vi "WFDC Compute Z Calibration.vi"(0 "Scan Positions File Name":string="Scan Positions.xml", 1 "User Close?":bool=TRUE, 2 "Half Shift":i32=7, 7 "Data Path":path, 11 "Error":errorcluster) -> (4 "Fit Slope":dbl=0.02 format="%#_6f", 8 "Fit Intercept":dbl=0.02, 13 "Ref Images":T1[](array[typedef]), 15 "Error":errorcluster)   [LabVIEW 2016]
uses:
  <vilib>/vision/Image Controls.llb/IMAQ Image.ctl
  WFDC Controls/WFDC Reference Image Info.ctl
  <vilib>/Utility/miscctls.llb/LVPointTypeDef.ctl
  <vilib>/Analysis/6fits.llb/Curve Fitting Criteria.ctl
  WFDC DLL and Testing/Visual Studio NCC Max Shift DLL/x64/Release/VSmaxShiftNCC.dll
  <vilib>/Analysis/NI_AALPro.lvlib
panel:
  out "Z Calibration":cluster{dbl[], dbl[]}[](graph)
  in  "Done":bool
  out "Wait Bar":i32(slide) scale=0.0..11.0
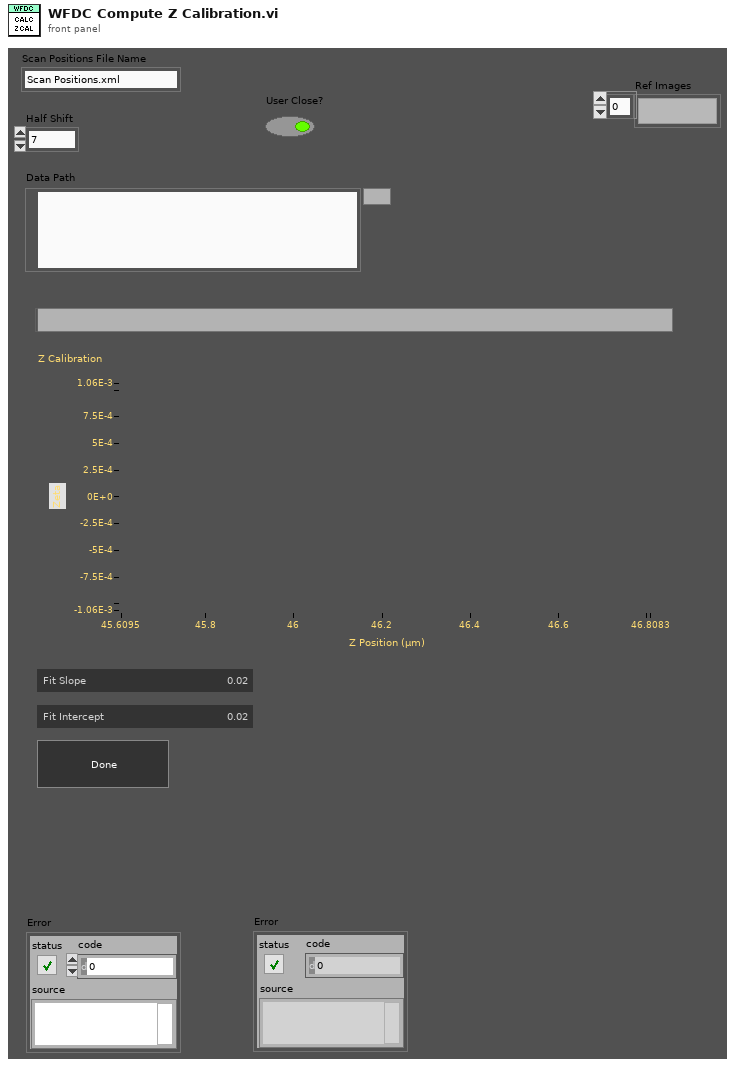
[diagram p1: front panel]
types:
  T1 = typedef "IMAQ Image.ctl" = refnum<image>
  T2 = enum16{"Always On", "Always Off", "Off While Running"}
  T3 = typedef "LVPointTypeDef.ctl" = cluster{"Horizontal":i16, "Vertical":i16}
  T4 = typedef "WFDC Reference Image Info.ctl" = cluster{"Image Path":path, "Z Position":dbl, "Number of Frames":u32}
  T5 = typedef "LVRectTypeDef.ctl" = cluster{"Left":i16, "Top":i16, "Right":i16, "Bottom":i16}
  T6 = typedef "LVBoundsTypeDef.ctl" = cluster{"Width":u32, "Height":u32}
  T7 = typedef "NI_AALPro.lvlib/Curve Fitting Criteria.ctl" = u16
  T8 = typedef "TIF Read Image Information.ctl" = cluster{"Byte Order":enum16{"big-endian, network order", "native, host order", "little-endian"}, "Width (pixels)":i32, "Height (pixels)":i32, "Bits per Pixel":u8, "Total Frames":u32, "First Frame Offset (bytes)":u32, "Frame Size (bytes)":u32}
  T9 = typedef "Image Type" = u32
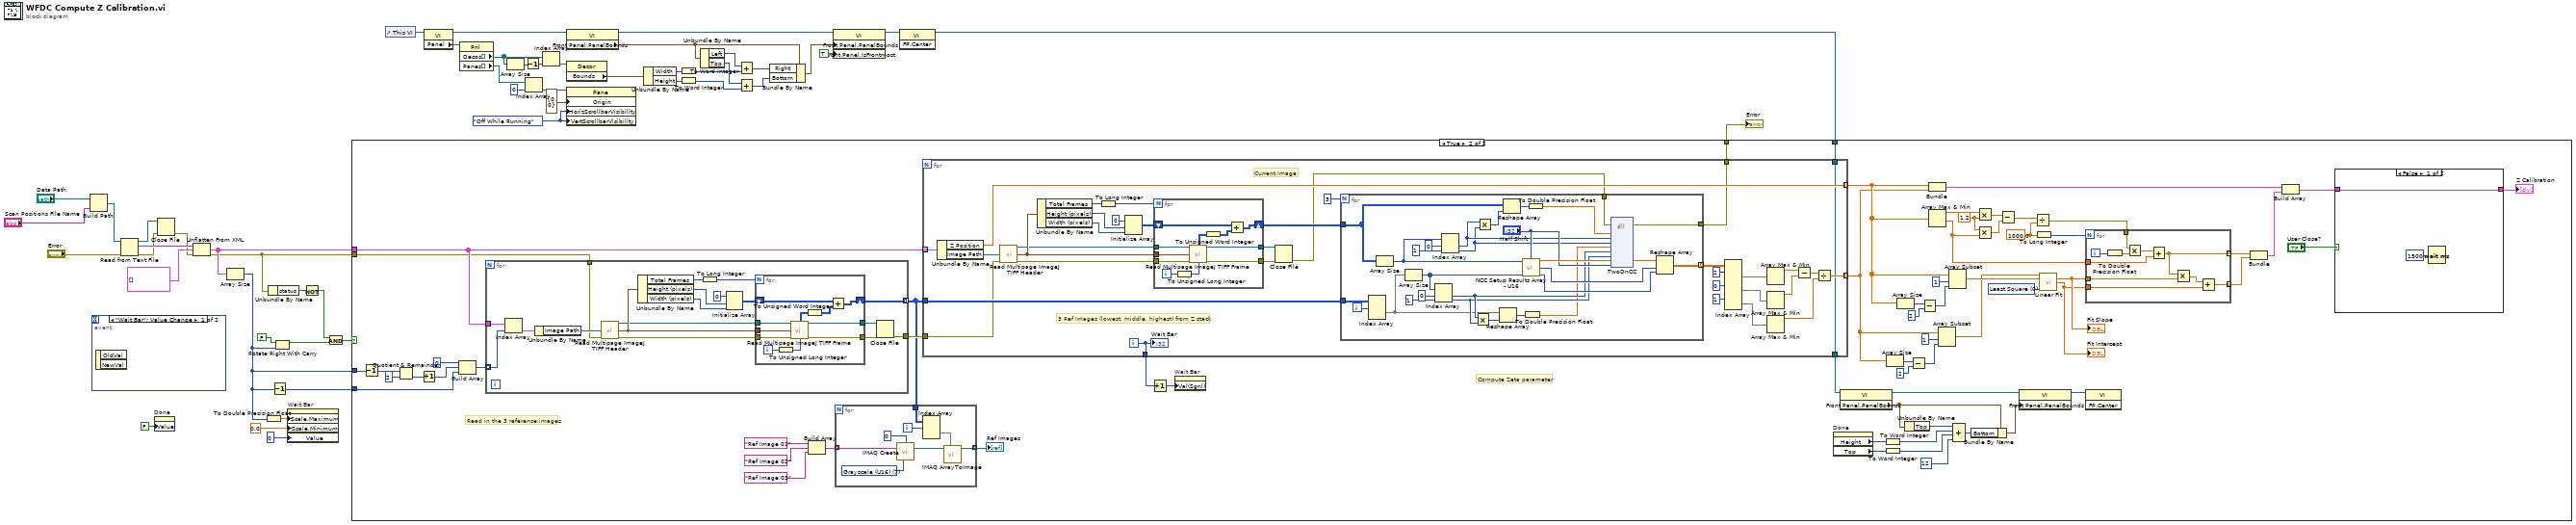
[diagram p0: block diagram]
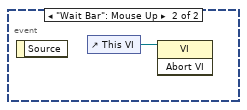
[diagram p2: hidden frame]
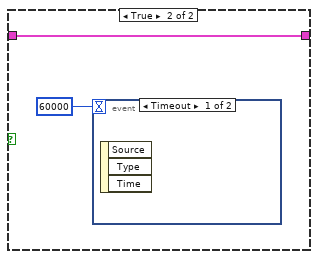
[diagram p4: hidden frame]
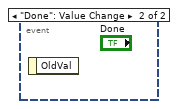
[diagram p5: hidden frame]
diagram:
  w25 = T2."Off While Running" ("Vertical Scrollbar Visibility")
  n1 = Build Path(base path="Data Path", name or relative path="Scan Positions File Name") -> (appended path=w1:path)
  n2 = event shown="[0] \"Wait Bar\": Value Change" {
    selector: _ -> [_ _]
    dyn-events: _ -> [_ _]
    timeout: _ -> [_ _]
    event "Wait Bar": Value Change {
      n3 = event-data() -> ()  [unwired: 1 in, 2 out]
    }
    event "Wait Bar": Mouse Up {
      n4 = event-data() -> ()  [unwired: 1 in, 1 out]
      n5 = control-ref of="This VI"() -> (w51:refnum<vi>)
      n6 = invoke class="VI" method="Abort VI"(reference=w51) -> ()  [unwired: 2 in, 3 out]
    }
  }
  n7 = Read from Text File(file (use dialog)=w1, error in="Error") -> (refnum out=w49:refnum<file>, text=w50:string, error out=w44:errorcluster)  [unwired: 2 in, 1 out]
  n8 = property on="Done" class="Bool (strict)"("Value"=FALSE ("Done")) -> ()  [unwired: 2 in, 2 out]
  n9 = Close File(refnum=w49, error in=w44) -> (error out=w43:errorcluster)  [unwired: 1 out]
  n10 = Unflatten From XML(xml string=w50, type=T4[] [], error in (no error)=w43) -> (value=w46:T4[], error out=w42:errorcluster)
  n11 = Array Size(array=w46) -> (size(s)=w9:i32)
  n12 = To Double Precision Float(number=w9) -> (double precision float=w8:dbl)
  n13 = Unbundle By Name(w42) -> ("status"=w41:bool)
  n14 = Decrement(x=w9) -> (x-1=w45:i32)
  n15 = Rotate Right With Carry(2:w9, 3:FALSE ("carry")) -> (1:w39:bool)  [unwired: 1 out]
  n16 = property on="Wait Bar" class="Slide (strict)"("Scale.Maximum"=w8, "Scale.Minimum"=0.0 ("Scale.Range:Minimum"), "Value"=0 ("Wait Bar")) -> ()  [unwired: 2 in, 2 out]
  n17 = Not(x=w41) -> (.not. x?=w40:bool)
  n18 = And(x=w40, y=w39) -> (x .and. y?=w38:bool)
  n19 = control-ref of="This VI"() -> (w12:refnum<vi>)
  n20 = property class="VI"(reference=w12) -> (reference out=w26:refnum<vi>, "Panel"=w19:refnum<vi>)  [unwired: 1 in, 1 out]
  n21 = property class="Pnl"(reference=w19) -> ("Decos[]"=w18:refnum<vi>[], "Panes[]"=w22:refnum<vi>[])  [unwired: 1 in, 2 out]
  n22 = Array Size(array=w18) -> (size(s)=w16:i32)
  n23 = Decrement(x=w16) -> (x-1=w17:i32)
  n24 = Index Array(array=w22, index=0) -> (element=w21:refnum<vi>)
  n25 = Index Array(array=w18, index=w17) -> (element=w24:refnum<vi>)
  n26 = property class="VI"(reference=w26) -> (reference out=w28:refnum<vi>, "Front Panel.PanelBounds"=w29:T5)  [unwired: 1 in, 1 out]
  n27 = property class="Decor"(reference=w24) -> ("Bounds"=w27:T6)  [unwired: 1 in, 2 out]
  n28 = property class="Pane"(reference=w21, "Origin"=T3 {"Horizontal"=0, "Vertical"=0}, "HorizScrollbarVisibility"=w25, "VertScrollbarVisibility"=w25) -> ()  [unwired: 1 in, 2 out]
  n29 = Unbundle By Name(w27) -> ("Width"=w32:u32, "Height"=w35:u32)
  n30 = To Word Integer(number=w32) -> (16bit integer=w34:i16)
  n31 = To Word Integer(number=w35) -> (16bit integer=w13:i16)
  n32 = Unbundle By Name(w29) -> ("Left"=w31:i16, "Top"=w15:i16)
  n33 = Add(x=w31, y=w34) -> (x+y=w33:i16)
  n34 = Add(x=w15, y=w13) -> (x+y=w14:i16)
  n35 = Bundle By Name(cluster=w29, "Right"=w33, "Bottom"=w14) -> (w30:T5)
  n36 = property class="VI"(reference=w28, "Front Panel.PanelBounds"=w30, "Front Panel.IsFrontmost"=TRUE ("Front Panel Window:Is Frontmost")) -> (reference out=w5:refnum<vi>)  [unwired: 1 in, 1 out]
  n37 = invoke class="VI" method="FP.Center"(reference=w5) -> (reference out=w4:refnum<vi>)  [unwired: 2 in, 2 out]
  n38 = case shown="True" w38 {
    tunnel: w9 -> [_ w116]
    tunnel: w46 -> [_ w108]
    tunnel: w45 -> [_ w110]
    tunnel: w42 -> [w52 w81]
    tunnel: [w52 w79] -> w36
    tunnel: w4 -> [_ w74]
    frame False {
    }
    frame True {
      w101 = 1000.0 ("y")
      w105 = 1.2 ("y")
      w107 = T7 0 items=["Least Square", "Least Absolute Residual", "Bisquare"] ("method")
      # "Compute Zeta parameter"
      # "Read in the 3 reference images"
      n39 = Decrement(x=w116) -> (x-1=w115:i32)
      n40 = Quotient & Remainder(x=w115, y=2) -> (floor(x/y)=w113:i32)  [unwired: 1 out]
      n41 = Increment(x=w113) -> (x+1=w112:i32)
      n42 = Build Array(0 ("element"), w112, w110) -> (w109:i32[])
      n43 = for {
        tunnel: w109 -> [w228] mode=indexing
        tunnel: w108 -> [w229]
        tunnel: [w215] -> w60 mode=indexing
        tunnel: [w213] -> w80
        tunnel: w81 -> [w212]
        n44 = Index Array(array=w229, index=w228) -> (element=w227:T4)
        n45 = Unbundle By Name(w227) -> ("Image Path"=w216:path)
        n46 = call "Read Multipage ImageJ TIFF Header.vi"("TIFF Path"=w216, "Error"=w212) -> ("TIF Ref"=w218:refnum<file>, "Image Info"=w220:T8, "Error"=w219:errorcluster)  [unwired: 11 in]
        n47 = Unbundle By Name(w220) -> ("Total Frames"=w221:u32, "Height (pixels)"=w225:i32, "Width (pixels)"=w224:i32)
        n48 = To Long Integer(number=w221) -> (32bit integer=w222:i32)
        n49 = Initialize Array(u16 0 ("element"), w225, w224) -> (w223:u16[][])
        n50 = for {
          N: w222 -> [_]
          tunnel: w218 -> [w240]
          tunnel: w220 -> [w239]
          tunnel: w219 -> [w238]
          shift-right: [w234] -> w215
          shift-left: w223 -> [w235]
          tunnel: [w233] -> w226
          tunnel: [w232] -> w214
          i -> [w237]
          n51 = To Unsigned Long Integer(number=w237) -> (unsigned 32bit integer=w236:u32)
          n52 = call "Read Multipage ImageJ TIFF Frame.vi"("TIF Ref"=w240, "Image Info"=w239, "Error"=w238, "Frame"=w236) -> ("U8 Image"=w231:u8[][], "TIF Ref (Dup)"=w233:refnum<file>, "Error"=w232:errorcluster)  [unwired: 8 in, 1 out]
          n53 = To Unsigned Word Integer(number=w231) -> (unsigned 16bit integer=w230:u16[][])
          n54 = Add(x=w235, y=w230) -> (x+y=w234:u16[][])
        }
        n55 = Close File(refnum=w226, error in=w214) -> (error out=w213:errorcluster)  [unwired: 1 out]
      }
      n56 = Build Array("Ref Image 01" ("Image Name"), "Ref Image 02" ("Image Name"), "Ref Image 03" ("Image Name")) -> (w64:string[])
      n57 = for {
        tunnel: w64 -> [w126] mode=indexing
        tunnel: w60 -> [w124]
        tunnel: [w121] -> w59 mode=indexing
        i -> [w122]
        w127 = T9 7 items=["Grayscale (U8)", "Grayscale (I16)", "Grayscale (SGL)", "Complex (CSG)", "RGB (U32)", "HSL (U32)", "RGB (U64)", "Grayscale (U16)"] ("Image Type")
        n58 = call "IMAQ Create"("Border Size"=0, "Image Name"=w126, "Image Type"=w127) -> ("New Image"=w125:T1)  [unwired: 2 in, 1 out]
        n59 = Index Array(array=w124, index (dim 0)=w122) -> (element=w123:u16[][])  [unwired: 2 in]
        n60 = call "IMAQ ArrayToImage"("Image Pixels (U16)"=w123, "Image"=w125) -> ("Image Out"=w121:T1)  [unwired: 8 in, 1 out]
      }
      "Ref Images" <- w59
      n61 = for {
        tunnel: w60 -> [w172]
        tunnel: w108 -> [w171] mode=indexing
        tunnel: [w170] -> w83 mode=indexing
        tunnel: [w169] -> w82 mode=indexing
        tunnel: w80 -> [w168]
        tunnel: [w167] -> w79
        tunnel: [w166] -> w78
        tunnel: w74 -> [w165]
        tunnel: [w165] -> w73
        i -> [w166]
        # "Current Image"
        # "3 Ref Images (lowest, middle, highest) from Z stack"
        n62 = Unbundle By Name(w171) -> ("Z Position"=w170:dbl, "Image Path"=w154:path)
        n63 = call "Read Multipage ImageJ TIFF Header.vi"("TIFF Path"=w154, "Error"=w168) -> ("TIF Ref"=w156:refnum<file>, "Image Info"=w158:T8, "Error"=w157:errorcluster)  [unwired: 11 in]
        n64 = Unbundle By Name(w158) -> ("Total Frames"=w159:u32, "Height (pixels)"=w163:i32, "Width (pixels)"=w162:i32)
        n65 = To Long Integer(number=w159) -> (32bit integer=w160:i32)
        n66 = Initialize Array(u16 0 ("element"), w163, w162) -> (w161:u16[][])
        n67 = for {
          N: w160 -> [_]
          tunnel: w156 -> [w211]
          tunnel: w158 -> [w210]
          tunnel: w157 -> [w209]
          shift-right: [w205] -> w152
          shift-left: w161 -> [w206]
          tunnel: [w204] -> w164
          tunnel: [w203] -> w140
          i -> [w208]
          n68 = To Unsigned Long Integer(number=w208) -> (unsigned 32bit integer=w207:u32)
          n69 = call "Read Multipage ImageJ TIFF Frame.vi"("TIF Ref"=w211, "Image Info"=w210, "Error"=w209, "Frame"=w207) -> ("U8 Image"=w202:u8[][], "TIF Ref (Dup)"=w204:refnum<file>, "Error"=w203:errorcluster)  [unwired: 8 in, 1 out]
          n70 = To Unsigned Word Integer(number=w202) -> (unsigned 16bit integer=w201:u16[][])
          n71 = Add(x=w206, y=w201) -> (x+y=w205:u16[][])
        }
        n72 = Close File(refnum=w164, error in=w140) -> (error out=w139:errorcluster)  [unwired: 1 out]
        n73 = for {
          N: 3 -> [_]
          tunnel: w172 -> [w200]
          tunnel: w152 -> [w180]
          tunnel: [w175] -> w151 mode=indexing
          tunnel: w139 -> [w174]
          tunnel: [w173] -> w167
          i -> [w199]
          n74 = Index Array(array=w200, index (dim 0)=w199) -> (element=w187:u16[][])  [unwired: 2 in]
          n75 = Array Size(array=w180) -> (size(s)=w182:i32[])
          n76 = Array Size(array=w187) -> (size(s)=w193:i32[])
          n77 = Index Array(array=w193, index #1=0 ("index"), index #2=1 ("index")) -> (element #1=w190:i32, element #2=w189:i32)
          n78 = Index Array(array=w182, index #1=0 ("index"), index #2=1 ("index")) -> (element #1=w178:i32, element #2=w177:i32)
          n79 = Multiply(x=w190, y=w189) -> (x*y=w188:i32)
          n80 = Multiply(x=w178, y=w177) -> (x*y=w176:i32)
          n81 = Reshape Array(w187, w188) -> (w186:u16[])
          n82 = Reshape Array(w180, w176) -> (w181:u16[])
          n83 = call "NCC Setup Results Array - U16.vi"("Image 01 Size"=w182, "Half Shift"="Half Shift", "Image 02 Size"=w193) -> ("NCC Results Array"=w198:dbl[], "Result Rows"=w195:i32, "Result Columns"=w196:i32)  [unwired: 10 in]
          n84 = To Double Precision Float(number=w186) -> (double precision float=w185:dbl[])
          n85 = To Double Precision Float(number=w181) -> (double precision float=w179:dbl[])
          n86 = dll-call lib="C:/Users/George Sirinakis/Documents/Microscope-Control/Microscope Modules/Wide Field Drift Correction/WFDC DLL and Testing/Visual Studio NCC Max Shift DLL/x64/Release/VSmaxShiftNCC.dll" fn="TwoDnCC"(error in=w174, "im01"=w179, "im01rowSize"=w178, "im01colSize"=w177, "im02"=w185, "im02rowSize"=w190, "im02ColSize"=w189, "theResult"=w198, "halfShift"="Half Shift") -> (error out=w173:errorcluster, "theResult"=w197:dbl[])  [unwired: 10 in, 1 out]
          n87 = Reshape Array(w197, w195, w196) -> (w175:dbl[][])
        }
        n88 = Index Array(array=w151, index (dim 0) #1=2 ("index (page)"), index (dim 0) #2=0 ("index (page)"), index (dim 0) #3=1 ("index (page)")) -> (element #1=w143:dbl[][], element #2=w141:dbl[][], element #3=w142:dbl[][])  [unwired: 6 in]
        n89 = Array Max & Min(array=w143) -> (max value=w147:dbl)  [unwired: 3 out]
        n90 = Array Max & Min(array=w141) -> (max value=w146:dbl)  [unwired: 3 out]
        n91 = Array Max & Min(array=w142) -> (max value=w144:dbl)  [unwired: 3 out]
        n92 = Subtract(x=w147, y=w146) -> (x-y=w145:dbl)
        n93 = Divide(x=w145, y=w144) -> (x/y=w169:dbl)
        "Wait Bar" <- w166
      }
      n94 = Increment(x=w78) -> (x+1=w77:i32)
      n95 = property on="Wait Bar" class="Slide (strict)"("Val(Sgnl)"=w77) -> ()  [unwired: 2 in, 2 out]
      n96 = property on="Done" class="Bool (strict)"() -> ("Height"=w69:u32, "Top"=w68:i32)  [unwired: 2 in, 2 out]
      n97 = property class="VI"(reference=w73) -> (reference out=w75:refnum<vi>, "Front Panel.PanelBounds"=w72:T5)  [unwired: 1 in, 1 out]
      n98 = To Word Integer(number=w69) -> (16bit integer=w67:i16)
      n99 = To Word Integer(number=w68) -> (16bit integer=w66:i16)
      n100 = Array Size(array=w82) -> (size(s)=w92:i32)
      n101 = Array Size(array=w83) -> (size(s)=w89:i32)
      n102 = Unbundle By Name(w72) -> ("Top"=w71:i16)
      n103 = Subtract(x=w92, y=2) -> (x-y=w90:i32)
      n104 = Subtract(x=w89, y=2) -> (x-y=w88:i32)
      n105 = Bundle(w83, w82) -> (w95:cluster{dbl[], dbl[]})  [unwired: 1 in]
      n106 = Array Max & Min(array=w83) -> (max value=w106:dbl, min value=w99:dbl)  [unwired: 2 out]
      n107 = Array Subset(array=w82, index=1, length=w90) -> (w84:dbl[])
      n108 = Array Subset(array=w83, index=1, length=w88) -> (w85:dbl[])
      n109 = Compound Arithmetic op=ADD(w71, w67, w66, i16 12) -> (w70:i16)
      n110 = Bundle By Name(cluster=w72, "Bottom"=w70) -> (w76:T5)
      n111 = Multiply(x=w106, y=w105) -> (x*y=w104:dbl)
      n112 = Multiply(x=w105, y=w99) -> (x*y=w103:dbl)
      n113 = Subtract(x=w104, y=w103) -> (x-y=w102:dbl)
      n114 = property class="VI"(reference=w75, "Front Panel.PanelBounds"=w76) -> (reference out=w58:refnum<vi>)  [unwired: 1 in, 1 out]
      n115 = Divide(x=w102, y=w101) -> (x/y=w98:dbl)
      n116 = To Long Integer(number=w101) -> (32bit integer=w100:i32)
      n117 = call <vilib>:"Linear Fit.vi"("Y"=w84, "X"=w85, "method"=w107) -> ("slope"=w57:dbl, "intercept"=w56:dbl)  [unwired: 8 in, 3 out]
      "Fit Slope" <- w57
      "Fit Intercept" <- w56
      n118 = for {
        N: w100 -> [_]
        tunnel: w99 -> [w134]
        tunnel: w98 -> [w136]
        tunnel: [w133] -> w97 mode=indexing
        tunnel: w56 -> [w130]
        tunnel: w57 -> [w132]
        tunnel: [w129] -> w96 mode=indexing
        i -> [w138]
        n119 = To Double Precision Float(number=w138) -> (double precision float=w137:dbl)
        n120 = Multiply(x=w136, y=w137) -> (x*y=w135:dbl)
        n121 = Add(x=w135, y=w134) -> (x+y=w133:dbl)
        n122 = Multiply(x=w133, y=w132) -> (x*y=w131:dbl)
        n123 = Add(x=w131, y=w130) -> (x+y=w129:dbl)
      }
      n124 = invoke class="VI" method="FP.Center"(reference=w58) -> ()  [unwired: 2 in, 3 out]
      n125 = Bundle(w97, w96) -> (w94:cluster{dbl[], dbl[]})  [unwired: 1 in]
      n126 = Build Array(w95, w94) -> (w55:cluster{dbl[], dbl[]}[])
      n127 = case shown="False" "User Close?" {
        tunnel: w55 -> [w117 w119]
        tunnel: [w117 w119] -> w54
        frame False {
          n128 = Wait (ms)(milliseconds to wait=u32 1500) -> ()  [unwired: 1 out]
        }
        frame True {
          n129 = event shown="[0] Timeout" {
            selector: _ -> [_ _]
            dyn-events: _ -> [_ _]
            timeout: 60000 -> [_ _]
            event Timeout {
              n130 = event-data() -> ()  [unwired: 1 in, 3 out]
            }
            event "Done": Value Change {
              n131 = event-data() -> ()  [unwired: 1 in, 1 out]
            }
          }
        }
      }
      "Z Calibration" <- w54
    }
  }
  "Error" <- w36
